vi "DFD Cascade Filters.vi"(8 "error in (no error)":errorcluster, 9 "filters in":T1[](array[typedef]) {"mSRate_QSettings"."source" items=["Coef a/k"=0, "Coef b/v"=7, "Input"=1, "Output"=2, "Multiplicand"=3, "Product"=4, "Sum"=5, "Delay"=6, "Gain"=8]}, 10 "filter in 2":T1={"mSRate_Fs"=1.0, "mSRate_Version"="2.0", "mSRate_Comments"="", "mSRate_OrgCoef"={"type"=enum."Undefined", "gain"=1.0, "coef a (k)"=[], "coef b (v)"=[]}, "mSRate_CurCoef"={"type"=enum."Undefined", "gain"=1.0, "coef a (k)"=[], "coef b (v)"=[]}, "mSRate_Quantized?"=FALSE, "mSRate_QCoef"={"type"=enum."Undefined", "gain"=1.0, "coef a (k)"=[], "coef b (v)"=[]}, "mSRate_QSettings"=[], "mSRate_Order"=0, "mSRate_Scaling"={"mSRate_ScaleByPowerOf2?"=FALSE, "mSRate_ScaleType"=enum."No Norm"}} {"mSRate_QSettings"."source" items=["Coef a/k"=0, "Coef b/v"=7, "Input"=1, "Output"=2, "Multiplicand"=3, "Product"=4, "Sum"=5, "Delay"=6, "Gain"=8]}, 11 "filter in 1":T1={"mSRate_Fs"=1.0, "mSRate_Version"="2.0", "mSRate_Comments"="", "mSRate_OrgCoef"={"type"=enum."Undefined", "gain"=1.0, "coef a (k)"=[], "coef b (v)"=[]}, "mSRate_CurCoef"={"type"=enum."Undefined", "gain"=1.0, "coef a (k)"=[], "coef b (v)"=[]}, "mSRate_Quantized?"=FALSE, "mSRate_QCoef"={"type"=enum."Undefined", "gain"=1.0, "coef a (k)"=[], "coef b (v)"=[]}, "mSRate_QSettings"=[], "mSRate_Order"=0, "mSRate_Scaling"={"mSRate_ScaleByPowerOf2?"=FALSE, "mSRate_ScaleType"=enum."No Norm"}} {"mSRate_QSettings"."source" items=["Coef a/k"=0, "Coef b/v"=7, "Input"=1, "Output"=2, "Multiplicand"=3, "Product"=4, "Sum"=5, "Delay"=6, "Gain"=8]}) -> (0 "error out":errorcluster, 3 "filter out":T1={"mSRate_Fs"=1.0, "mSRate_Version"="2.0", "mSRate_Comments"="", "mSRate_OrgCoef"={"type"=enum."Undefined", "gain"=1.0, "coef a (k)"=[], "coef b (v)"=[]}, "mSRate_CurCoef"={"type"=enum."Undefined", "gain"=1.0, "coef a (k)"=[], "coef b (v)"=[]}, "mSRate_Quantized?"=FALSE, "mSRate_QCoef"={"type"=enum."Undefined", "gain"=1.0, "coef a (k)"=[], "coef b (v)"=[]}, "mSRate_QSettings"=[], "mSRate_Order"=0, "mSRate_Scaling"={"mSRate_ScaleByPowerOf2?"=FALSE, "mSRate_ScaleType"=enum."No Norm"}} {"mSRate_QSettings"."source" items=["Coef a/k"=0, "Coef b/v"=7, "Input"=1, "Output"=2, "Multiplicand"=3, "Product"=4, "Sum"=5, "Delay"=6, "Gain"=8]})   [LabVIEW 2017, in "NI_DigFilterLicensed.lvlib"]
doc: "Creates a new filter by cascading two or more filters."
uses:
  <vilib>/addons/Digital Filter Design/NI_DigFilterLicensed.lvlib
  <vilib>/addons/Digital Filter Design/_Objects.llb/DFD Filter Obj.ctl
  <vilib>/addons/Digital Filter Design/_Objects.llb/DFD Filter Coef.ctl
  <vilib>/addons/Digital Filter Design/_Objects.llb/DFD Filter Structure Type Selector.ctl
  <vilib>/addons/Digital Filter Design/_Objects.llb/dfd_Internal Quantization Settings.ctl
  <vilib>/addons/Digital Filter Design/_Objects.llb/dfd_Internal Quantization Srcs.ctl
  <vilib>/addons/Digital Filter Design/_Objects.llb/DFD Coef Norm Type.ctl
  <vilib>/Analysis/2dsp.llb/1D Convolution (DBL).vi
  <vilib>/Analysis/NI_AALPro.lvlib
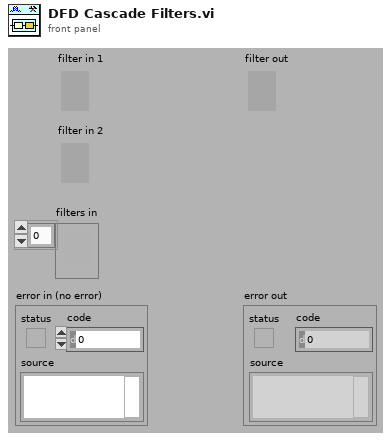
[diagram p1: front panel]
types:
  T1 = typedef "NI_DigFilterLicensed.lvlib/DFD Filter Obj.ctl" = cluster{"mSRate_Fs":dbl, "mSRate_Version":string, "mSRate_Comments":string, "mSRate_OrgCoef":T2, "mSRate_CurCoef":T2, "mSRate_Quantized?":bool, "mSRate_QCoef":T2, "mSRate_QSettings":T4[], "mSRate_Order":i32, "mSRate_Scaling":cluster{"mSRate_ScaleByPowerOf2?":bool, "mSRate_ScaleType":T6}}
  T2 = typedef "NI_DigFilterLicensed.lvlib/DFD Filter Coef.ctl" = cluster{"type":T3, "gain":dbl, "coef a (k)":dbl[], "coef b (v)":dbl[]}
  T3 = typedef "NI_DigFilterLicensed.lvlib/DFD Filter Structure Type Selector.ctl" = enum16{"Undefined", "FIR Direct Form", "FIR Direct Form Transposed", "FIR Symmetric", "FIR Antisymmetric", "IIR Direct Form I", "IIR Direct Form I Transposed", "IIR Direct Form II", "IIR Direct Form II Transposed", "IIR Cascaded Second Order Sections Form I", "IIR Cascaded Second Order Sections Form I Transposed", "IIR Cascaded Second Order Sections Form II", "IIR Cascaded Second Order Sections Form II Transposed", "Lattice Allpass (basic sections)", "Lattice Allpass (one multiplier sections)", "Lattice Allpass (normalized sections)", "Lattice AR (basic sections)", "Lattice AR (one multiplier sections)", "Lattice AR (normalized sections)", "Lattice MA (minimum phase)", "Lattice MA (maximum phase)", "Lattice ARMA (basic sections)", "Lattice ARMA (one multiplier sections)", "Lattice ARMA (normalized sections)"}
  T4 = typedef "NI_DigFilterLicensed.lvlib/dfd_Internal Quantization Settings.ctl" = cluster{"source":T5, "wl":i16, "iwl":i16, "overflow mode":enum16{"Saturation", "Wrap"}, "rounding mode":enum16{"Nearest", "Truncation"}, "signed?":bool}
  T5 = typedef "NI_DigFilterLicensed.lvlib/dfd_Internal Quantization Srcs.ctl" = u16
  T6 = typedef "NI_DigFilterLicensed.lvlib/DFD Coef Norm Type.ctl" = enum16{"No Norm", "Time Domain 1-Norm", "Time Domain 2-Norm", "Time Domain Inf-Norm"}
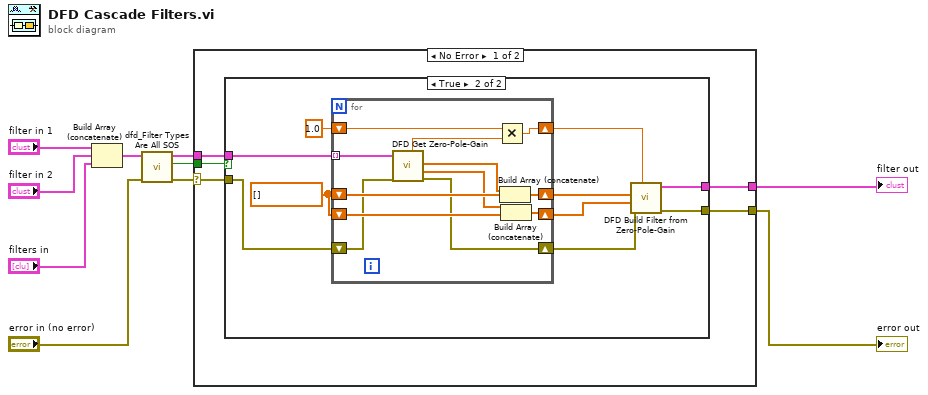
[diagram p0: block diagram]
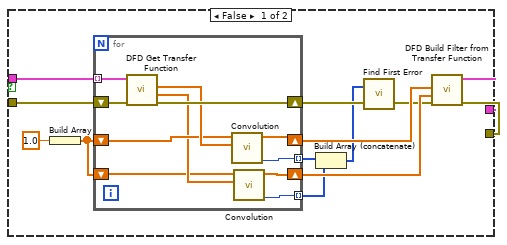
[diagram p2: hidden frame]
diagram:
  n1 = Build Array (concatenate)("filter in 1", "filter in 2", "filters in") -> (w4:T1[])
  n2 = call <vilib>:"dfd_Filter Types Are All SOS.vi"("error in (no error)"="error in (no error)", "filters in"=w4) -> ("error out"=w1:errorcluster, "All SOS?"=w3:bool, "filters out"=w2:T1[])  [unwired: 7 out]
  n3 = case shown="No Error" w1 {
    selector: w1 -> [w11 w62]
    tunnel: [w15 w62] -> w9
    tunnel: [w14 _] -> w5
    tunnel: w3 -> [w13 _]
    tunnel: w2 -> [w12 _]
    frame No Error {
      n4 = case shown="True" w13 {
        tunnel: w12 -> [w28 w49]
        tunnel: w11 -> [w27 w48]
        tunnel: [w25 w40] -> w14
        tunnel: [w24 w41] -> w15
        frame False {
          n5 = Build Array(1.0) -> (w20:dbl[])
          n6 = for {
            tunnel: w28 -> [w39] mode=indexing
            shift-right: [w37] -> w26
            shift-left: w27 -> [w38]
            shift-right: [w34] -> w23
            shift-left: w20 -> [w35]
            shift-right: [w31] -> w22
            shift-left: w20 -> [w32]
            tunnel: [w30] -> w18 mode=indexing
            tunnel: [w29] -> w17 mode=indexing
            n7 = call <vilib>:"DFD Get Transfer Function.vi"("error in (no error)"=w38, "filter in"=w39) -> ("error out"=w37:errorcluster, "denominator"=w33:dbl[], "numerator"=w36:dbl[])  [unwired: 7 out]
            n8 = call-poly <vilib>:"Convolution.vi"("Y"=w36, "X"=w35) -> ("error"=w30:i32, "X * Y"=w34:dbl[])  [unwired: 1 in, 7 out]
            n9 = call-poly <vilib>:"Convolution.vi"("Y"=w33, "X"=w32) -> ("error"=w29:i32, "X * Y"=w31:dbl[])  [unwired: 1 in, 7 out]
          }
          n10 = Build Array (concatenate)(w18, w17) -> (w16:i32[])
          n11 = call <vilib>:"Find First Error.vi"("error in (no error)"=w26, "error codes"=w16) -> ("error out"=w19:errorcluster)  [unwired: 1 in, 2 out]
          n12 = call <vilib>:"DFD Build Filter from Transfer Function.vi"("error in (no error)"=w19, "denominator"=w22, "numerator"=w23) -> ("error out"=w24:errorcluster, "filter out"=w25:T1)  [unwired: 2 in, 5 out]
        }
        frame True {
          w47 = cdb[] []
          n13 = for {
            tunnel: w49 -> [w56] mode=indexing
            shift-right: [w52] -> w42
            shift-left: w48 -> [w53]
            shift-right: [w58] -> w44
            shift-left: w47 -> [w59]
            shift-right: [w61] -> w45
            shift-left: w47 -> [w60]
            shift-right: [w57] -> w43
            shift-left: 1.0 -> [w51]
            n14 = call <vilib>:"DFD Get Zero-Pole-Gain.vi"("error in (no error)"=w53, "filter in"=w56) -> ("error out"=w52:errorcluster, "poles"=w54:cdb[], "zeroes"=w55:cdb[], "gain"=w50:dbl)  [unwired: 6 out]
            n15 = Multiply(x=w51, y=w50) -> (x*y=w57:dbl)
            n16 = Build Array (concatenate)(w55, w60) -> (w61:cdb[])
            n17 = Build Array (concatenate)(w54, w59) -> (w58:cdb[])
          }
          n18 = call <vilib>:"DFD Build Filter from Zero-Pole-Gain.vi"("gain"=w43, "error in (no error)"=w42, "poles"=w44, "zeroes"=w45) -> ("error out"=w41:errorcluster, "filter out"=w40:T1)  [unwired: 1 in, 5 out]
        }
      }
    }
    frame Error {
    }
  }
  "filter out" <- w5
  "error out" <- w9
